vi "Extract Excel Data 2010.vi"() -> ()   [LabVIEW 2011]
panel:
  out "data":string[][](array[string])
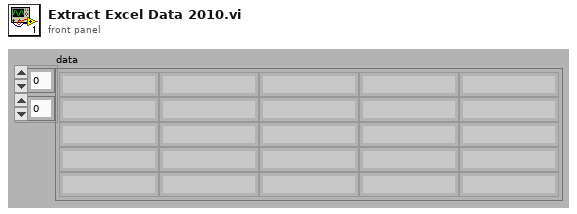
[diagram p1: front panel]
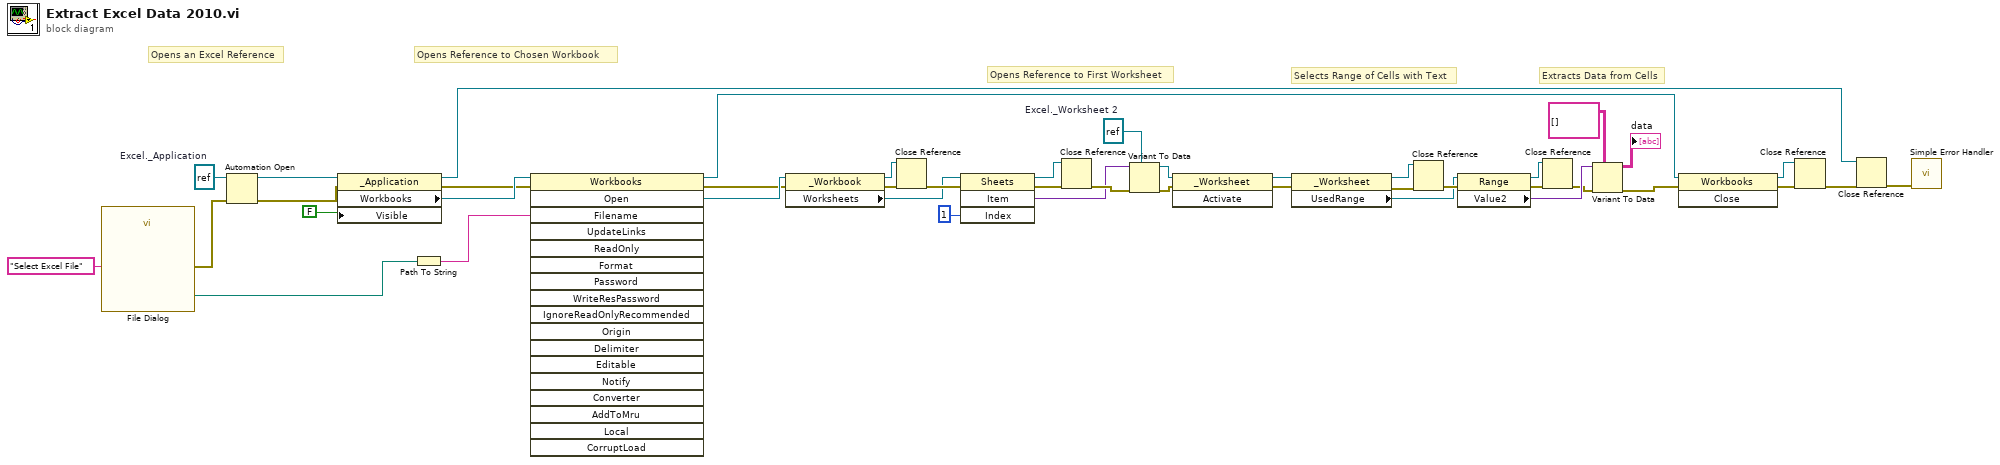
[diagram p0: block diagram]
diagram:
  w9 = refnum<k7> refnum  # Excel._Application
  w34 = refnum<k7> refnum  # Excel._Worksheet 2
  # "Opens an Excel Reference"
  # "Extracts Data from Cells"
  # "Selects Range of Cells with Text"
  # "Opens Reference to First Worksheet"
  # "Opens Reference to Chosen Workbook"
  n1 = call "File Dialog"("prompt"="Select Excel File") -> ("selected path"=w3:path, "error out"=w1:errorcluster)  [unwired: 11 in, 2 out]
  n2 = Automation Open(error in (no error)=w1, Automation Refnum=w9) -> (Automation Refnum=w8:refnum<k7>, error out=w7:errorcluster)  [unwired: 2 in]
  n3 = property class="_Application"(reference=w8, error in=w7, "Visible"=FALSE) -> (reference out=w4:refnum<k7>, error out=w10:errorcluster, "Workbooks"=w42:refnum<k7>)
  n4 = Path To String(path=w3) -> (string=w41:string)
  n5 = invoke class="Workbooks" method="Open"(reference=w42, error in=w10, "Filename"=w41) -> (reference out=w14:refnum<k7>, error out=w13:errorcluster, "Open"=w35:refnum<k7>)  [unwired: 15 in, 15 out]
  n6 = property class="_Workbook"(reference=w35, error in=w13) -> (reference out=w38:refnum<k7>, error out=w39:errorcluster, "Worksheets"=w37:refnum<k7>)
  n7 = Close Reference(reference=w38, error in (no error)=w39) -> (error out=w40:errorcluster)
  n8 = invoke class="Sheets" method="Item"(reference=w37, error in=w40, "Index"=1) -> (reference out=w31:refnum<k7>, error out=w33:errorcluster, "Item"=w30:variant)  [unwired: 1 in, 1 out]
  n9 = Close Reference(reference=w31, error in (no error)=w33) -> (error out=w32:errorcluster)
  n10 = Variant To Data(error in=w32, type=w34, Variant=w30) -> (data=w26:refnum<k7>, error out=w27:errorcluster)
  n11 = invoke class="_Worksheet" method="Activate"(reference=w26, error in=w27) -> (reference out=w22:refnum<k7>, error out=w21:errorcluster)  [unwired: 1 in, 1 out]
  n12 = property class="_Worksheet"(reference=w22, error in=w21) -> (reference out=w17:refnum<k7>, error out=w18:errorcluster, "UsedRange"=w16:refnum<k7>)
  n13 = Close Reference(reference=w17, error in (no error)=w18) -> (error out=w19:errorcluster)
  n14 = property class="Range"(reference=w16, error in=w19) -> (reference out=w29:refnum<k7>, error out=w24:errorcluster, "Value2"=w28:variant)
  n15 = Close Reference(reference=w29, error in (no error)=w24) -> (error out=w23:errorcluster)
  n16 = Variant To Data(error in=w23, type=string[][] [] ("Array"), Variant=w28) -> (data=→"data":string[][], error out=w15:errorcluster)
  n17 = invoke class="Workbooks" method="Close"(reference=w14, error in=w15) -> (reference out=w11:refnum<k7>, error out=w12:errorcluster)  [unwired: 1 in, 1 out]
  n18 = Close Reference(reference=w11, error in (no error)=w12) -> (error out=w6:errorcluster)
  n19 = Close Reference(reference=w4, error in (no error)=w6) -> (error out=w5:errorcluster)
  n20 = call <vilib>:"Simple Error Handler.vi"("error in (no error)"=w5) -> ()  [unwired: 4 in, 5 out]
